vi "HAL camera quit.vi"   [LabVIEW 2011]
uses:
  ixon1024/HAL Camera specifications globals.vi
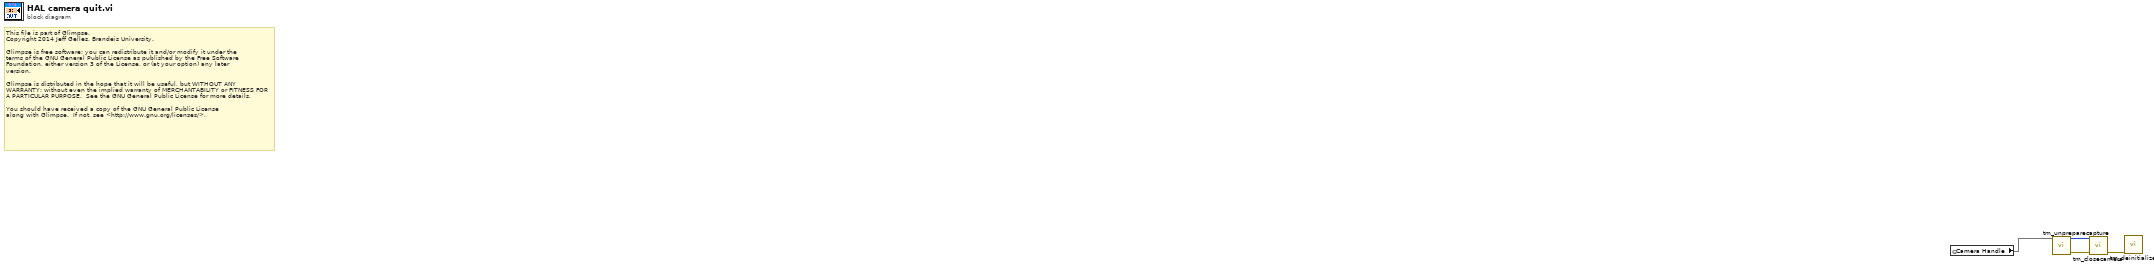
[diagram p0: block diagram]
diagram:
  # "This file is part of Glimpse. \nCopyright 2014 Jeff Gelles, Brandeis University.    \n\nGlimpse is free software: you can redistribute it and/or modify it under the \nterms of the GNU General Public License as published by the Free Software \nFoundation, either version 3 of the License, or (at your option) any later \nversion.\n\nGlimpse is distributed in the hope that it will be useful, but WITHOUT ANY \nWARRANTY; without even the implied warranty of MERCHANTABILITY or FITNESS FOR \nA PARTICULAR PURPOSE.  See the GNU General Public License for more details.\n\nYou should have received a copy of the GNU General Public License\nalong with Glimpse.  If not, see <http://www.gnu.org/licenses/>."
  n1 = global read "HAL Camera specifications globals.vi" "Camera Handle"() -> (w4)
  n2 = call <userlib>:"tm_unpreparecapture.vi"("Handle in"=w4) -> ("error out"=w2:errorcluster, "Handle out"=w3:u32)  [unwired: 9 in]
  n3 = call <userlib>:"tm_closecamera.vi"("error in (no error)"=w2, "Handle in"=w3) -> ("error out"=w1:errorcluster)  [unwired: 9 in]
  n4 = call <userlib>:"tm_deinitialize.vi"("error in (no error)"=w1) -> ()  [unwired: 10 in, 1 out]
